vi "Set Matrix - stdin.vi"(8 "error in":errorcluster, 9 "value":dbl[][](array[numeric]), 10 "variable name":string, 11 "pipe in":T1) -> (0 "error out":errorcluster, 3 "pipe out":T1)   [LabVIEW 2013, in "GOLPI library.lvlib"]
uses:
  GOLPI library.lvlib
  LV Process.lvlibp/Pipe Handle.ctl
  Globals.vi
  LV Process.lvlibp
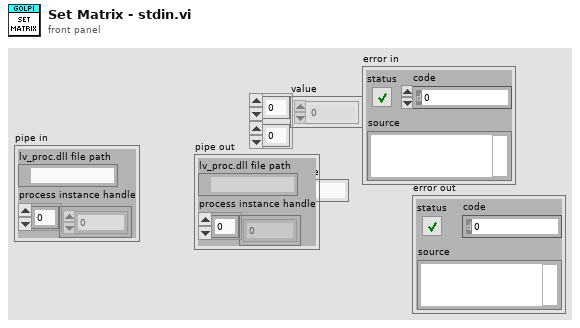
[diagram p1: front panel]
types:
  T1 = typedef "LV Process.lvlibp/Pipe Handle.ctl" = cluster{"lv_proc.dll file path":path, "process instance handle":u32[]}
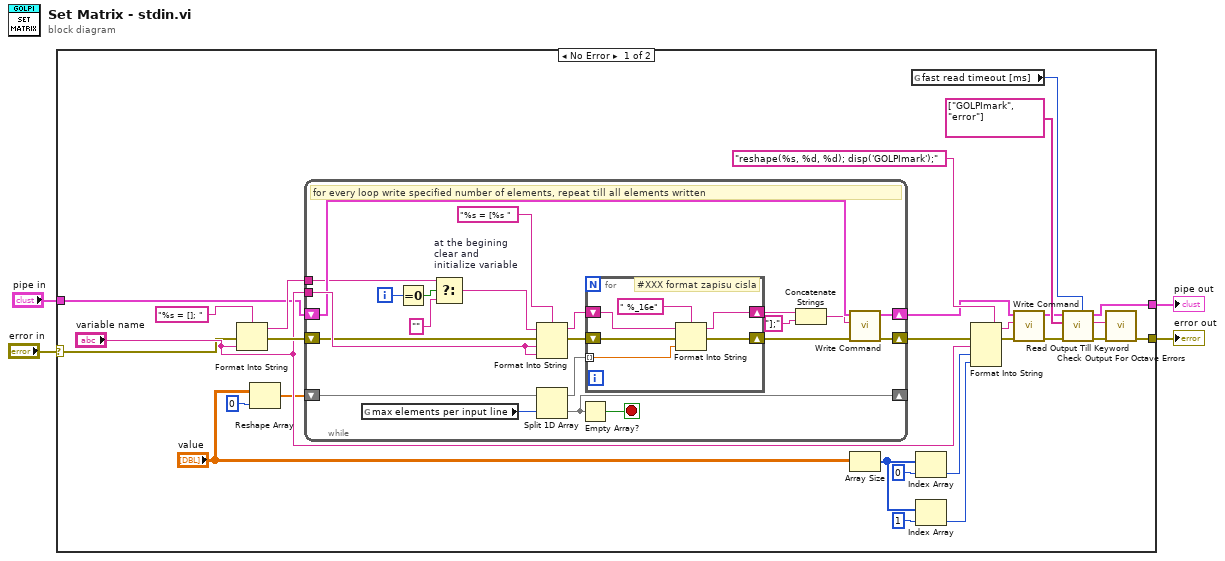
[diagram p0: block diagram]
diagram:
  n1 = case shown="No Error" "error in" {
    selector: "error in" -> [w7 w61]
    tunnel: [w8 w61] -> w4
    tunnel: "pipe in" -> [w6 w60]
    tunnel: [w5 w60] -> w1
    frame No Error {
      n2 = Format Into String(format string="%s = []; ", error in=w7, "variable name") -> (resulting string=w18:string, error out=w30:errorcluster)  [unwired: 1 in]
      n3 = Reshape Array("value", 0 ("dimension size")) -> (w20:dbl[])
      n4 = while {
        shift-right: [w51] -> _
        shift-left: w20 -> [w53]
        tunnel: "variable name" -> [w44]
        shift-right: [w40] -> w31
        shift-left: w30 -> [w43]
        shift-right: [w39] -> w15
        shift-left: w6 -> [w38]
        tunnel: w18 -> [w34]
        i -> [w36]
        stop <- w50 stop-if-true
        # "for every loop write specified number of elements, repeat till all elements written"
        n5 = global read "Globals.vi" "max elements per input line"() -> (w52:u32)
        n6 = Equal To 0?(x=w36) -> (x = 0?=w35:bool)
        n7 = Select "at the begining\nclear and\ninitialize variable"(t=w34, s=w35, f="") -> (s? t:f=w33:string)
        n8 = Format Into String(format string="%s = [%s ", initial string=w33, error in=w43, w44, w44) -> (resulting string=w47:string, error out=w42:errorcluster)
        n9 = Split 1D Array(array=w53, index=w52) -> (first subarray=w48:dbl[], second subarray=w51:dbl[])
        n10 = Empty Array?(array=w51) -> (empty?=w50:bool)
        n11 = for {
          tunnel: w48 -> [w59] mode=indexing
          shift-right: [w57] -> w46
          shift-left: w47 -> [w56]
          shift-right: [w54] -> w41
          shift-left: w42 -> [w55]
          # "#XXX format zapisu cisla"
          n12 = Format Into String(format string=" %_16e", initial string=w56, error in=w55, w59) -> (resulting string=w57:string, error out=w54:errorcluster)
        }
        n13 = Concatenate Strings(w46, "];" ("string")) -> (w37:string)
        n14 = call "Write Command.vi"("error in"=w41, "command"=w37, "pipe in"=w38) -> ("error out"=w40:errorcluster, "pipe out"=w39:T1)  [unwired: 7 in]
      }
      n15 = Array Size(array="value") -> (size(s)=w25:i32[])
      n16 = global read "Globals.vi" "fast read timeout [ms]"() -> (w11:u32)
      n17 = Index Array(array=w25, index=0) -> (element=w28:i32)
      n18 = Index Array(array=w25, index=1) -> (element=w29:i32)
      n19 = Format Into String(format string="reshape(%s, %d, %d); disp('GOLPImark');", error in=w31, "variable name", w28, w29) -> (resulting string=w17:string, error out=w16:errorcluster)  [unwired: 1 in]
      n20 = call "Write Command.vi"("error in"=w16, "command"=w17, "pipe in"=w15) -> ("error out"=w10:errorcluster, "pipe out"=w9:T1)  [unwired: 7 in]
      n21 = call "Read Output Till Keyword.vi"("timeout [ms]"=w11, "error in"=w10, "keywords"=string[] ["GOLPImark", "error"], "pipe in"=w9) -> ("error out"=w14:errorcluster, "read buffer"=w12:string, "pipe out"=w5:T1)  [unwired: 4 in, 1 out]
      n22 = call "Check Output For Octave Errors.vi"("error in"=w14, "read buffer"=w12) -> ("error out"=w8:errorcluster)  [unwired: 9 in]
    }
    frame Error {
    }
  }
  "error out" <- w4
  "pipe out" <- w1
